vi "Init Channel.vi"() -> (3 "Channel Data":T1)   [LabVIEW 2020, in "Flex.lvlib"]
uses:
  Flex.lvlib
  Channel Data.ctl
  Element.ctl
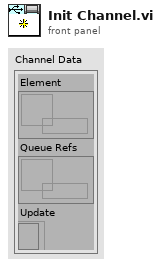
[diagram p1: front panel]
types:
  T1 = typedef "Flex.lvlib/Channel Data.ctl" = cluster{"Element":refnum<data-value>, "Queue Refs":refnum<data-value>, "Update":refnum<k4>}
  T2 = typedef "Flex.lvlib/Element.ctl" = dbl
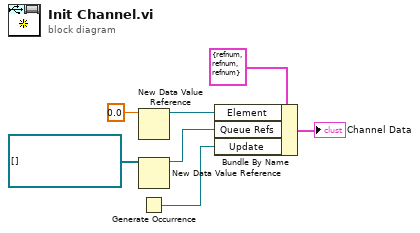
[diagram p0: block diagram]
diagram:
  n1 = New Data Value Reference(data value=T2 0.0 ("element")) -> (data value reference=w4:refnum<data-value>)  [unwired: 1 in, 1 out]
  n2 = New Data Value Reference(data value=refnum<queue>[] [] ("appended array")) -> (data value reference=w2:refnum<data-value>)  [unwired: 1 in, 1 out]
  n3 = Generate Occurrence() -> (w1:refnum<k4>)
  n4 = Bundle By Name(cluster=T1 {"Element"=refnum, "Queue Refs"=refnum, "Update"=refnum} ("Channel Data"), "Element"=w4, "Queue Refs"=w2, "Update"=w1) -> (→"Channel Data":T1)
